vi "getRightData_DriveQuadTalonSRX.vi"() -> (0 "Raw encoder counts R":dbl, 1 "Applied Output R":dbl format="%.5f", 2 "Encoder Velocity Units in 100ms R":dbl format="%.5f", 3 "Target Velocity Units in 100ms R":dbl format="%.5f", 4 "Distance FT R":dbl format="%.5f", 5 "Speed FT/SEC R":dbl format="%.5f", 7 "Speed Dmd FT/SEC R":dbl format="%.5f")   [LabVIEW 2019, in "DriveQuadTalonSRX_Motor.lvlib"]
uses:
  DriveQuadTalonSRX_Motor.lvlib
  globals_DriveQuadTalonSRX.vi
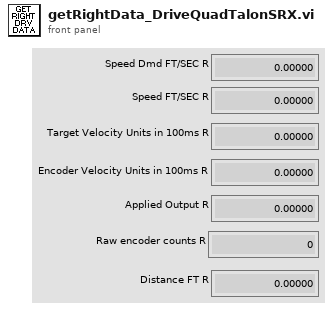
[diagram p1: front panel]
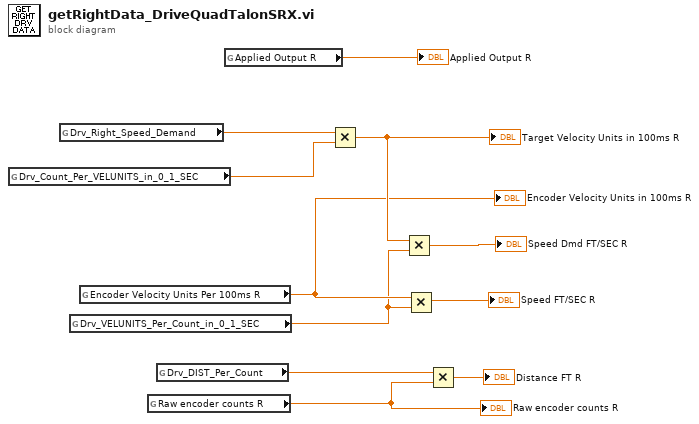
[diagram p0: block diagram]
diagram:
  n1 = global read "globals_DriveQuadTalonSRX.vi" "Drv_Count_Per_VELUNITS_in_0_1_SEC"() -> (w3:dbl)
  n2 = global read "globals_DriveQuadTalonSRX.vi" "Drv_Right_Speed_Demand"() -> (w7:dbl)
  n3 = global read "globals_DriveQuadTalonSRX.vi" "Drv_VELUNITS_Per_Count_in_0_1_SEC"() -> (w1:dbl)
  n4 = global read "globals_DriveQuadTalonSRX.vi" "Encoder Velocity Units Per 100ms R"() -> (w4:dbl)
  "Encoder Velocity Units in 100ms R" <- w4
  n5 = global read "globals_DriveQuadTalonSRX.vi" "Raw encoder counts R"() -> (w5:dbl)
  "Raw encoder counts R" <- w5
  n6 = global read "globals_DriveQuadTalonSRX.vi" "Drv_DIST_Per_Count"() -> (w2:dbl)
  n7 = global read "globals_DriveQuadTalonSRX.vi" "Applied Output R"() -> (→"Applied Output R":dbl)
  n8 = Multiply(x=w7, y=w3) -> (x*y=w8:dbl)
  "Target Velocity Units in 100ms R" <- w8
  n9 = Multiply(x=w8, y=w1) -> (x*y=→"Speed Dmd FT/SEC R":dbl)
  n10 = Multiply(x=w4, y=w1) -> (x*y=→"Speed FT/SEC R":dbl)
  n11 = Multiply(x=w2, y=w5) -> (x*y=→"Distance FT R":dbl)
